vi "acceptCommand.vi"(8 "error in (no error)":errorcluster, 11 "ElectrometerController in":refnum<class "ElectrometerController.lvclass">) -> (0 "error out":errorcluster, 3 "ElectrometerController out":refnum<class "ElectrometerController.lvclass">)   [LabVIEW 2016, in "ElectrometerController.lvclass"]
uses:
  ElectrometerController.lvclass
  ts_electrometeruserevents/Typedefs/CommandValue.ctl
  ElectrometerController.lvclass/ElectrometerController.ctl
  ts_electrometeruserevents/PubSubDataEvent/PubSubDataEvent.lvclass
  ts_electrometeruserevents/Typedefs/ElectrometerTypedefs.lvlib
  InternalCommandId/InternalCommandId.lvclass
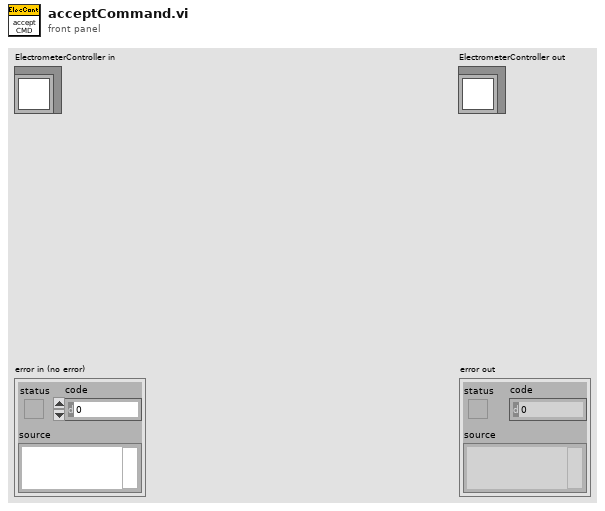
[diagram p1: front panel]
types:
  T1 = typedef "ElectrometerTypedefs.lvlib/CommandValue.ctl" = enum16{"N/A", "Disable", "Enable", "Exit", "GoToStandby", "OnHeartbeat", "OnIncomingMessagingError", "OnInterrupt", "Start", "SetDigitalFilter", "StartScan", "StartScanDt", "StartScanReachIntensity", "StopScan", "SetIntegrationTime", "PerformZeroCalib", "SetRange", "SetMode", "Power"}
  T2 = cluster{"error":i32, "result":string, "ack":i32, "cmdSeqNum":i32, "CommandValue":T1}
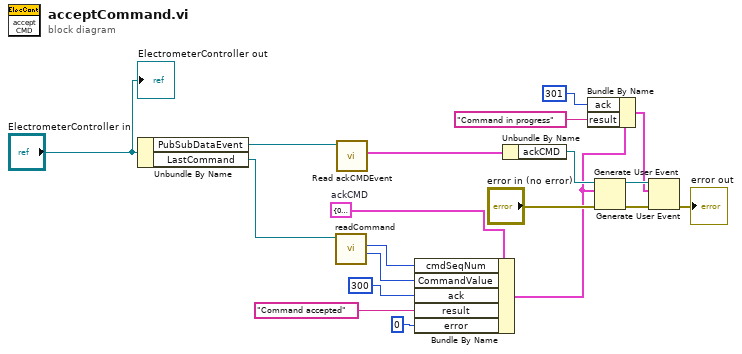
[diagram p0: block diagram]
diagram:
  w14 = T2 {"error"=0, "result"="", "ack"=0, "cmdSeqNum"=0, "CommandValue"=enum."N/A"}  # ackCMD
  n1 = Unbundle By Name("ElectrometerController in") -> ("PubSubDataEvent"=w13:refnum<class "PubSubDataEvent.lvclass">, "LastCommand"=w3:refnum<class "InternalCommandId.lvclass">)
  n2 = call "readCommand.vi"("InternalCommandId in"=w3) -> ("CommandValue"=w1:T1, "CommandID"=w2:i32)  [unwired: 7 in, 2 out]
  n3 = call-dynamic "Read ackCMDEvent.vi"("PubSubDataEvent in"=w13) -> ("ackCMDEvent"=w18:cluster{"ackCMD":refnum<user-event>})  [unwired: 8 in, 2 out]
  n4 = Bundle By Name(cluster=w14, "cmdSeqNum"=w2, "CommandValue"=w1, "ack"=300, "result"="Command accepted", "error"=0) -> (w8:T2)
  n5 = Unbundle By Name(w18) -> ("ackCMD"=w19:refnum<user-event>)
  n6 = Bundle By Name(cluster=w8, "ack"=301, "result"="Command in progress") -> (w5:T2)
  n7 = Generate User Event(user event=w19, event data cluster=w8, error in="error in (no error)") -> (user event out=w7:refnum<user-event>, error out=w10:errorcluster)  [unwired: 1 in]
  n8 = Generate User Event(user event=w7, event data cluster=w5, error in=w10) -> (error out=→"error out":errorcluster)  [unwired: 1 in, 1 out]
  "ElectrometerController out" <- "ElectrometerController in"
